vi "Handle Frame.vi"(8 "error in (no error)":errorcluster, 9 "Timeout ms":i32, 10 "Frame In":T1, 11 "WebsocketStream in":refnum<class "WebsocketStream.lvclass">) -> (0 "error out":errorcluster, 1 "Remaining  Timeout":i32, 3 "WebsocketStream out":refnum<class "WebsocketStream.lvclass">, 4 "Done?":bool)   [LabVIEW 2020, in "Stream-Websocket.lvlib" / "WebsocketStream.lvclass"]
uses:
  WebsocketStream.lvclass
  OpCode.ctl
  Stream-Websocket.lvlib
  Message Frame.ctl
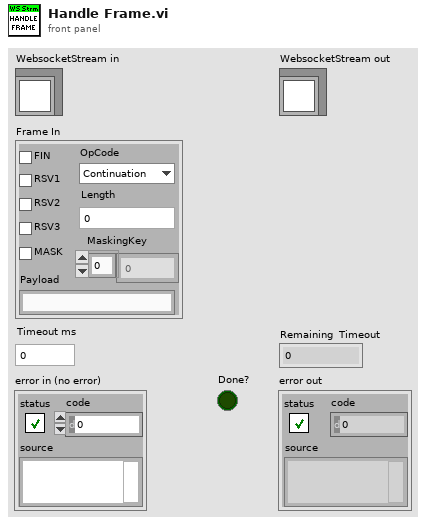
[diagram p1: front panel]
types:
  T1 = typedef "Stream-Websocket.lvlib/Message Frame.ctl" = cluster{"FIN":bool, "RSV1":bool, "RSV2":bool, "RSV3":bool, "MASK":bool, "OpCode":T2, "Length":u64, "MaskingKey":u8[], "Payload":string}
  T2 = typedef "Stream-Websocket.lvlib/OpCode.ctl" = enum8{"Continuation", "Text", "Binary", "Reserved3", "Reserved4", "Reserved5", "Reserved6", "Reserved7", "Close", "Ping", "Pong", "ReservedB", "ReservedC", "ReservedD", "ReservedE", "ReservedF"}
  T3 = typedef "Stream-Websocket.lvlib/WebsocketStream.lvclass/Ref Data.ctl" = cluster{"Command Queue":refnum<queue>, "Closing":bool}
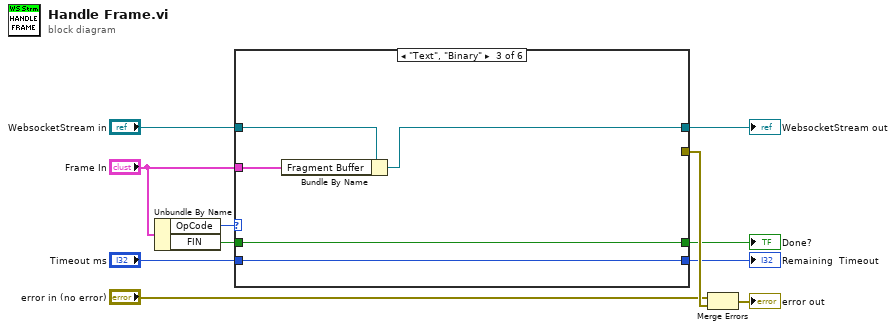
[diagram p0: block diagram]
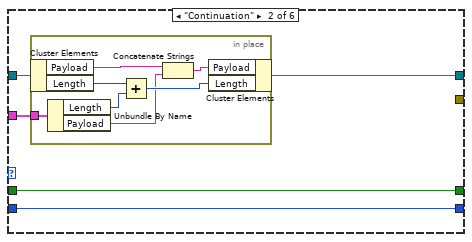
[diagram p3: hidden frame]
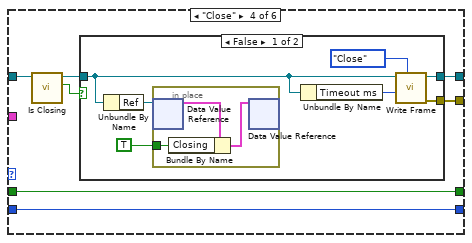
[diagram p4: hidden frame]
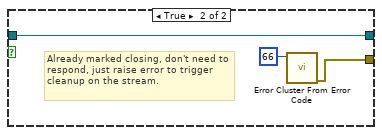
[diagram p5: hidden frame]
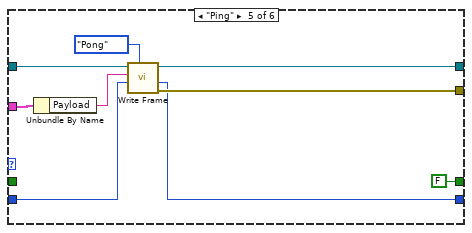
[diagram p6: hidden frame]
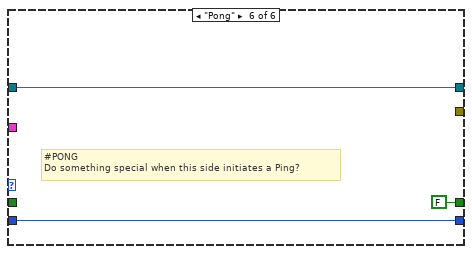
[diagram p7: hidden frame]
diagram:
  n1 = Unbundle By Name("Frame In") -> ("OpCode"=w10:T2, "FIN"=w8:bool)
  n2 = case shown="\"Text\", \"Binary\"" w10 {
    tunnel: "Frame In" -> [_ w16 w31 _ w58 _]
    tunnel: "WebsocketStream in" -> [w12 w17 w30 w37 w60 w62]
    tunnel: w8 -> [w13 w18 w29 w32 _ _]
    tunnel: "Timeout ms" -> [w14 w19 w27 w38 w56 w63]
    tunnel: [w13 w18 w29 w32 FALSE ("FIN") FALSE ("FIN")] -> w6
    tunnel: [w12 w15 w28 w34 w53 w62] -> w5
    tunnel: [w14 w19 w27 w38 w54 w63] -> w4
    tunnel: [_ _ _ w33 w55 _] -> w11
    frame Default {
    }
    frame "Continuation" {
      n3 = in-place {
        in-place-border: w16 -> [w26]
        n4 = in-place-cluster #1(w17) -> ("Payload"=w22:string, "Length"=w25:u64)
        n5 = Unbundle By Name(w26) -> ("Length"=w24:u64, "Payload"=w21:string)
        n6 = Add(x=w25, y=w24) -> (x+y=w23:u64)
        n7 = Concatenate Strings(w22, w21) -> (w20:string)
        n8 = in-place-cluster #1("Payload"=w20, "Length"=w23) -> (w15:refnum<class "WebsocketStream.lvclass">)
      }
    }
    frame "Text", "Binary" {
      n9 = Bundle By Name(cluster=w30, "Fragment Buffer"=w31) -> (w28:refnum<class "WebsocketStream.lvclass">)
    }
    frame "Close" {
      n10 = call "Is Closing.vi"("WebsocketStream in"=w37) -> ("Is Closing?"=w35:bool, "WebsocketStream out"=w36:refnum<class "WebsocketStream.lvclass">)  [unwired: 8 in, 1 out]
      n11 = case shown="False" w35 {
        tunnel: w36 -> [w40 w51]
        tunnel: [w44 w51] -> w34
        tunnel: [w43 w49] -> w33
        frame False {
          n12 = Unbundle By Name(w40) -> ("Ref"=w42:refnum<data-value>)
          n13 = in-place {
            in-place-border: TRUE -> [w46]
            n14 = in-place-dvr #2(w42) -> (w48:T3)  [unwired: 1 out]
            n15 = Bundle By Name(cluster=w48, "Closing"=w46) -> (w47:T3)
            n16 = in-place-dvr #2(w47) -> ()  [unwired: 2 out]
          }
          n17 = Unbundle By Name(w40) -> ("Timeout ms"=w39:i32)
          n18 = call "Write Frame.vi"("OpCode"=OpCode."Close", "Timeout ms"=w39, "WebsocketStream in"=w40) -> ("error out"=w43:errorcluster, "WebsocketStream out"=w44:refnum<class "WebsocketStream.lvclass">)  [unwired: 6 in, 1 out]
        }
        frame True {
          # "Already marked closing, don't need to respond, just raise error to trigger cleanup on the stream."
          n19 = call <vilib>:"Error Cluster From Error Code.vi"("error code (0)"=66) -> ("error out"=w49:errorcluster)  [unwired: 8 in]
        }
      }
    }
    frame "Ping" {
      n20 = Unbundle By Name(w58) -> ("Payload"=w57:string)
      n21 = call "Write Frame.vi"("OpCode"=OpCode."Pong", "Timeout ms"=w56, "Payload"=w57, "WebsocketStream in"=w60) -> ("error out"=w55:errorcluster, "Remaining  Timeout"=w54:i32, "WebsocketStream out"=w53:refnum<class "WebsocketStream.lvclass">)  [unwired: 5 in]
    }
    frame "Pong" {
      # "#PONG\nDo something special when this side initiates a Ping?"
    }
  }
  "WebsocketStream out" <- w5
  "Remaining  Timeout" <- w4
  "Done?" <- w6
  n22 = Merge Errors("error in (no error)", w11) -> (→"error out":errorcluster)
